vi "Write Value.vi"(8 "error in (no error)":errorcluster, 10 "Value":sgl, 11 "float in":refnum<class "float.lvclass">) -> (0 "error out":errorcluster, 3 "float out":refnum<class "float.lvclass">)   [LabVIEW 2020, in "Protobuf RAW.lvlib" / "float.lvclass"]
uses:
  float.lvclass
  float.lvclass/float.ctl
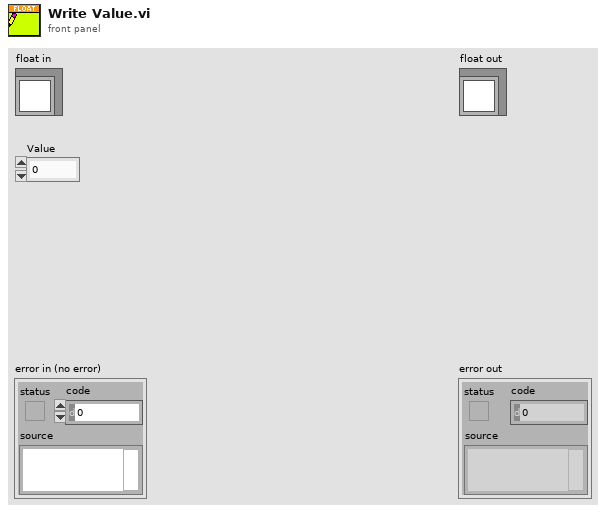
[diagram p1: front panel]
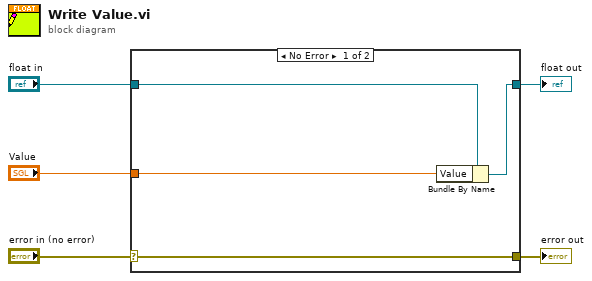
[diagram p0: block diagram]
diagram:
  n1 = case shown="No Error" "error in (no error)" {
    selector: "error in (no error)" -> [w9 w10]
    tunnel: [w9 w10] -> w4
    tunnel: [w7 w11] -> w2
    tunnel: "float in" -> [w8 w11]
    tunnel: "Value" -> [w6 _]
    frame No Error {
      n2 = Bundle By Name(cluster=w8, "Value"=w6) -> (w7:refnum<class "float.lvclass">)
    }
    frame Error {
    }
  }
  "error out" <- w4
  "float out" <- w2
